vi "ServerV2.vi"() -> ()   [LabVIEW 2021]
panel:
  out "BOK":u8(slide) scale=0.0..100.0
  out "kek":bool
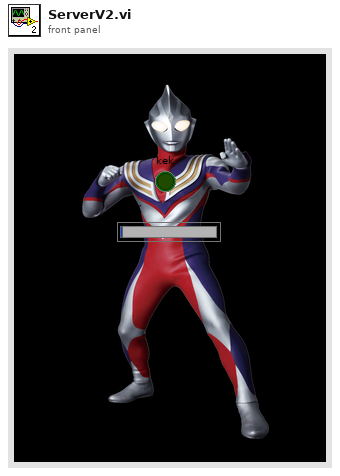
[diagram p1: front panel]
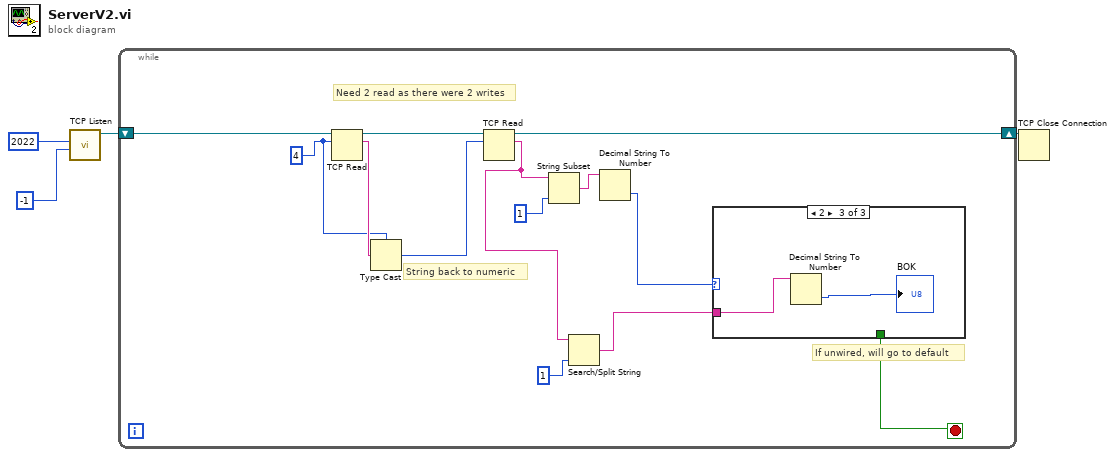
[diagram p0: block diagram]
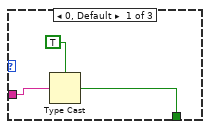
[diagram p2: hidden frame]
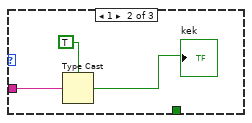
[diagram p3: hidden frame]
diagram:
  n1 = call <vilib>:"TCP Listen.vi"("timeout ms (wait forever: -1)"=-1, "port"=2022) -> ("connection ID"=w2:refnum<k5>)  [unwired: 5 in, 4 out]
  n2 = while {
    shift-right: [w15] -> w1
    shift-left: w2 -> [w17]
    stop <- w5 stop-if-true
    w13 = 4
    # "If unwired, will go to default"
    # "String back to numeric"
    # "Need 2 read as there were 2 writes"
    n3 = TCP Read(connection ID=w17, bytes to read=w13) -> (connection ID out=w16:refnum<k5>, data out=w14:string)  [unwired: 3 in, 1 out]
    n4 = Type Cast(type=w13, x=w14) -> (*(type *) &x=w12:i32)
    n5 = TCP Read(connection ID=w16, bytes to read=w12) -> (connection ID out=w15:refnum<k5>, data out=w8:string)  [unwired: 3 in, 1 out]
    n6 = String Subset(string=w8, length (rest)=1) -> (substring=w10:string)  [unwired: 1 in]
    n7 = Search/Split String(string=w8, offset (0)=1) -> (match + rest of string=w6:string)  [unwired: 1 in, 2 out]
    n8 = Decimal String To Number(string=w10) -> (number=w9:i32)  [unwired: 2 in, 1 out]
    n9 = case shown="2" w9 {
      tunnel: w6 -> [w19 w22 w25]
      tunnel: [w18 _ _] -> w5
      frame 0, Default {
        n10 = Type Cast(type=TRUE, x=w19) -> (*(type *) &x=w18:bool)
      }
      frame 1 {
        n11 = Type Cast(type=TRUE, x=w22) -> (*(type *) &x=→"kek":bool)
      }
      frame 2 {
        n12 = Decimal String To Number(string=w25) -> (number=→"BOK":i32)  [unwired: 2 in, 1 out]
      }
    }
  }
  n13 = TCP Close Connection(connection ID=w1) -> ()  [unwired: 2 in, 2 out]
